vi "Find Register Offset.vi"(8 "error in (no error)":errorcluster, 10 "register name":string, 11 "session in":u32) -> (0 "error out":errorcluster, 2 "resource offset":u32, 3 "session out":u32)   [LabVIEW 2026, in "FPGA Register IO.lvlib"]
uses:
  FPGA Register IO.lvlib
  TypeDefs/Register Data Store.ctl
  NiFpga.dll
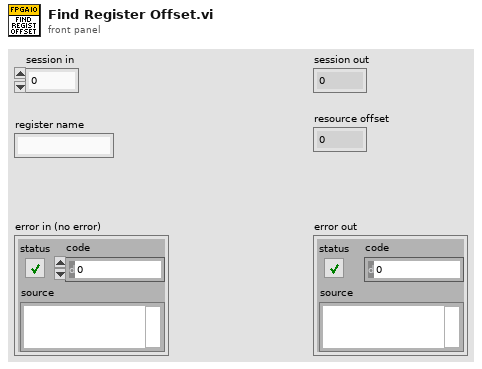
[diagram p1: front panel]
types:
  T1 = typedef "FPGA Register IO.lvlib/Register Data Store.ctl" = map{string, u32}
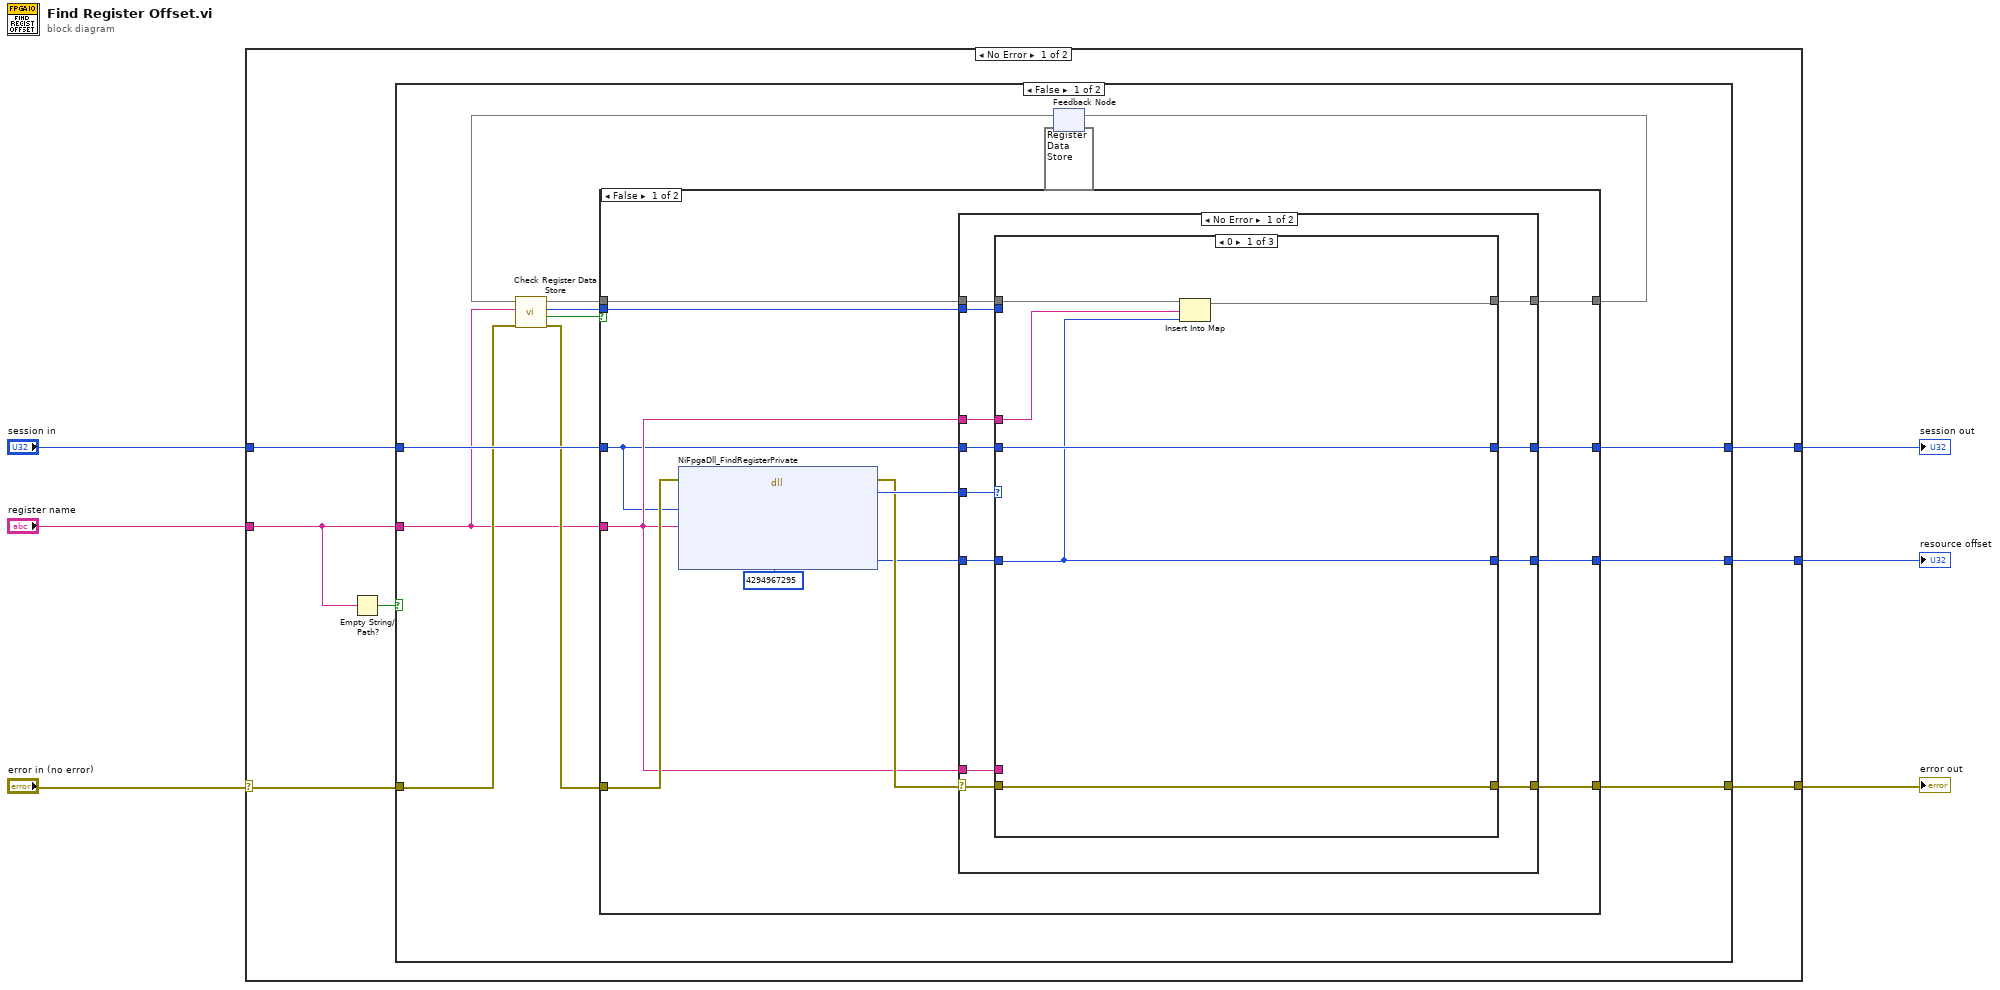
[diagram p0: block diagram]
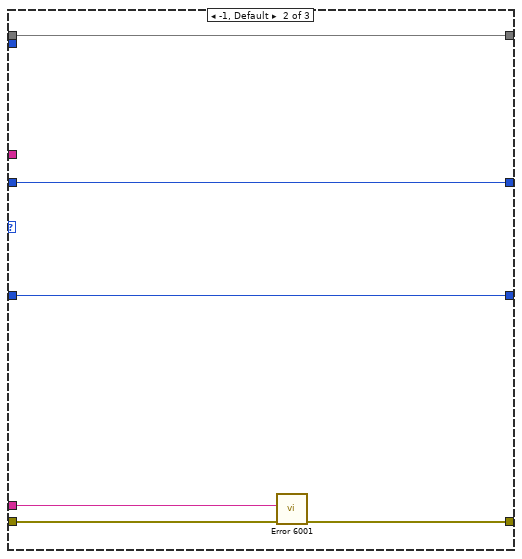
[diagram p2: hidden frame]
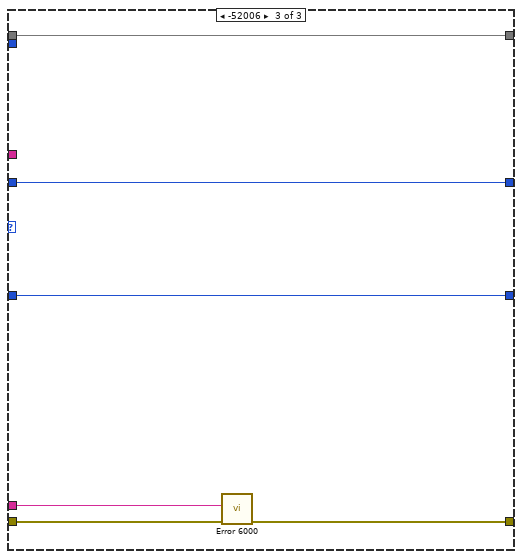
[diagram p3: hidden frame]
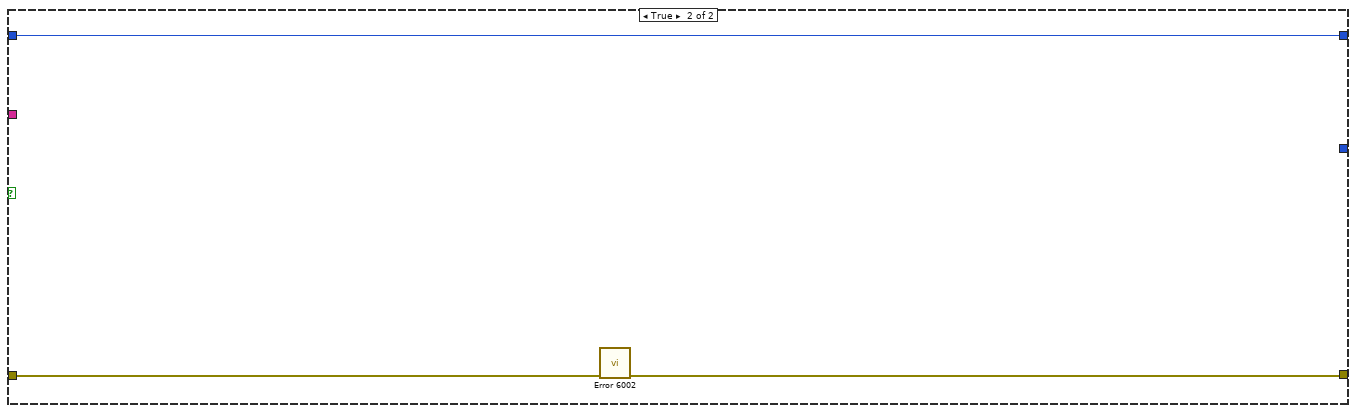
[diagram p6: hidden frame]
diagram:
  n1 = case shown="No Error" "error in (no error)" {
    selector: "error in (no error)" -> [w9 w82]
    tunnel: [w12 w82] -> w3
    tunnel: "register name" -> [w8 _]
    tunnel: "session in" -> [w13 w81]
    tunnel: [w11 w81] -> w4
    tunnel: [w10 _] -> w2
    frame No Error {
      n2 = Empty String/Path?(string/path=w8) -> (empty?=w7:bool)
      n3 = case shown="False" w7 {
        tunnel: w13 -> [w26 w78]
        tunnel: [w25 w79] -> w12
        tunnel: [w24 w78] -> w11
        tunnel: [w23 _] -> w10
        tunnel: w9 -> [w17 w80]
        tunnel: w8 -> [w14 _]
        frame False {
          n4 = feedback #1(T1 {}) -> (w21:T1)
          n5 = call "Check Register Data Store.vi"("error in (no error)"=w17, "register name"=w14, "register data store in"=w21) -> ("error IO"=w16:errorcluster, "Found"=w15:bool, "register offset"=w19:u32, "register data store out"=w20:T1)  [unwired: 5 in]
          n6 = case shown="False" w15 {
            tunnel: w16 -> [w38 w76]
            tunnel: w26 -> [w29 w77]
            tunnel: [w27 w74] -> w23
            tunnel: [w36 w76] -> w25
            tunnel: [w28 w77] -> w24
            tunnel: w14 -> [w32 _]
            tunnel: w20 -> [w34 w75]
            tunnel: w19 -> [w33 w74]
            tunnel: [w30 w75] -> w18
            frame False {
              n7 = dll-call lib="NiFpga.*" fn="NiFpgaDll_FindRegisterPrivate"(error in=w38, "session"=w29, "registerName"=w32, "expectedResourceType"=u32 4294967295) -> (error out=w35:errorcluster, "status"=w37:i32, "resourceOffset"=w31:u32)  [unwired: 6 in, 1 out]
              n8 = case shown="No Error" w35 {
                selector: w35 -> [w48 w73]
                tunnel: w37 -> [w51 _]
                tunnel: [w50 w73] -> w36
                tunnel: w32 -> [w49 _]
                tunnel: w34 -> [w47 w70]
                tunnel: w33 -> [w46 _]
                tunnel: w32 -> [w45 _]
                tunnel: w31 -> [w44 w71]
                tunnel: [w43 w70] -> w30
                tunnel: w29 -> [w42 w72]
                tunnel: [w41 w72] -> w28
                tunnel: [w40 w71] -> w27
                frame No Error {
                  n9 = case shown="0" w51 {
                    tunnel: [w57 w58 w69] -> w50
                    tunnel: w49 -> [_ w59 w64]
                    tunnel: w48 -> [w57 w60 w68]
                    tunnel: w47 -> [w55 w63 w66]
                    tunnel: w46 -> [_ _ _]
                    tunnel: w45 -> [w54 _ _]
                    tunnel: w44 -> [w53 w61 w65]
                    tunnel: [w52 w63 w66] -> w43
                    tunnel: w42 -> [w56 w62 w67]
                    tunnel: [w56 w62 w67] -> w41
                    tunnel: [w53 w61 w65] -> w40
                    frame 0 {
                      n10 = Insert Into Map(map in=w55, key=w54, value=w53) -> (map out=w52:T1)  [unwired: 2 out]
                    }
                    frame -1, Default {
                      n11 = call "Error 6001.vi"("error in (no error)"=w60, "register name"=w59) -> ("error out"=w58:errorcluster)  [unwired: 9 in]
                    }
                    frame -52006 {
                      n12 = call "Error 6000.vi"("error in (no error)"=w68, "register name"=w64) -> ("error out"=w69:errorcluster)  [unwired: 9 in]
                    }
                  }
                }
                frame Error {
                }
              }
            }
            frame True {
            }
          }
          n13 = feedback-in #1(w18) -> ()
        }
        frame True {
          n14 = call "Error 6002.vi"("error in (no error)"=w80) -> ("error out"=w79:errorcluster)  [unwired: 10 in]
        }
      }
    }
    frame Error {
    }
  }
  "session out" <- w4
  "error out" <- w3
  "resource offset" <- w2
